vi "niFpga Discrete Transfer Function Direct.vi"(7 "reset":bool, 10 "FXP Transfer Function Model":T1={"Numerator"=[0.0, 0.0, 0.0, 0.0, 0.0, 0.0, 0.0, 0.0, 0.0], "Denominator"=[0.0, 0.0, 0.0, 0.0, 0.0, 0.0, 0.0, 0.0, 0.0], "Order"=0}, 11 "input u(k)":fxp<+/-,32,16>) -> (3 "output y(k)":fxp<+/-,32,16>)   [LabVIEW 2017]
doc: "Implements a fixed-point transfer function system model on an FPGA. Obtain this model by using the Discrete FP Transfer Function to FXP VI."
uses:
  <vilib>/rvi/Analysis/control/linear/templates/niFPGA FXP Transfer Function Model.ctl
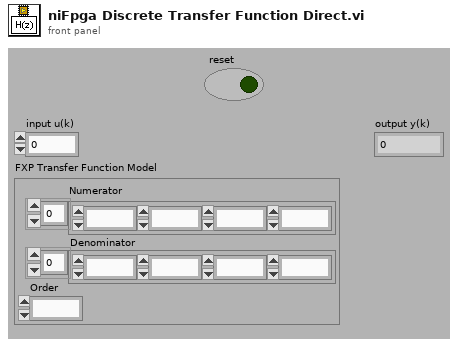
[diagram p1: front panel]
types:
  T1 = typedef "niFPGA FXP Transfer Function Model.ctl" = cluster{"Numerator":fxp<+/-,32,12>[], "Denominator":fxp<+/-,32,12>[], "Order":u8}
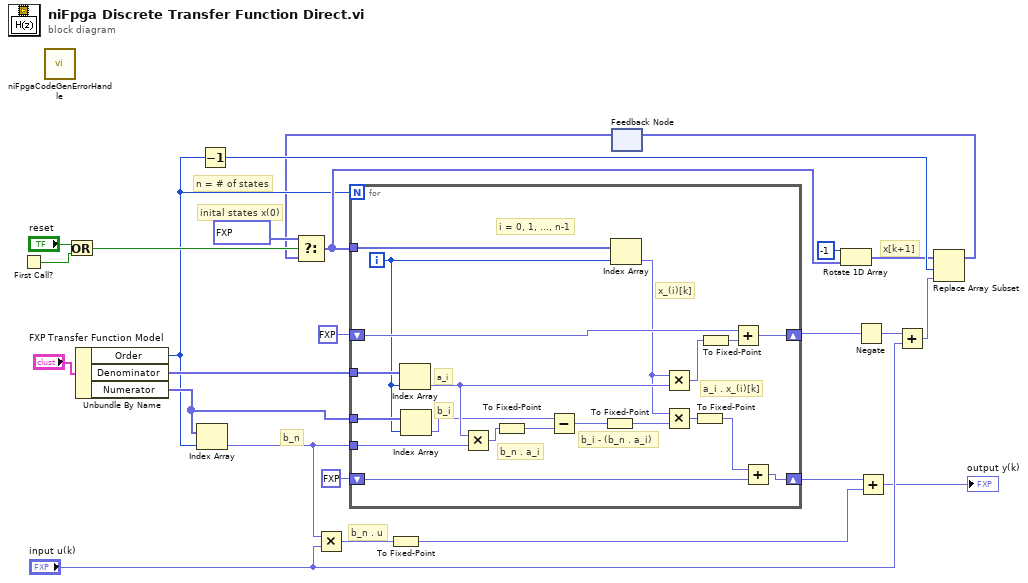
[diagram p0: block diagram]
diagram:
  # "b_n . u"
  # "b_n"
  # "x[k+1]"
  # "n = # of states"
  # "inital states x(0)"
  n1 = First Call?() -> (First Call?: T/F=w24:bool)
  n2 = call <vilib>:"niFpgaCodeGenErrorHandle.vi"() -> ()  [unwired: 1 in]
  n3 = Or(x="reset", y=w24) -> (x .or. y?=w23:bool)
  n4 = Unbundle By Name("FXP Transfer Function Model") -> ("Order"=w13:u8, "Denominator"=w14:fxp<+/-,32,12>[], "Numerator"=w19:fxp<+/-,32,12>[])
  n5 = Index Array(array=w19, index=w13) -> (element=w20:fxp<+/-,32,12>)
  n6 = Decrement(x=w13) -> (x-1=w17:u8)
  n7 = Multiply(x=w20, y="input u(k)") -> (x*y=w4:fxp<+/-,64,28>)
  n8 = To Fixed-Point(number=w4) -> (fixed-point=w3:fxp<+/-,32,16>)  [unwired: 1 in]
  n9 = feedback #1() -> (w12:fxp<+/-,32,16>[])  [unwired: 1 in]
  n10 = Select(t=fxp<+/-,32,16>[] [0.0, 0.0, 0.0, 0.0, 0.0, 0.0, 0.0, 0.0, 0.0] ("initialized array"), s=w23, f=w12) -> (s? t:f=w16:fxp<+/-,32,16>[])
  n11 = for {
    N: w13 -> [_]
    tunnel: w14 -> [w39]
    shift-right: [w44] -> w10
    shift-left: fxp<+/-,32,16> 0.0 ("element") -> [w45]
    tunnel: w19 -> [w38]
    tunnel: w20 -> [w43]
    shift-right: [w42] -> w7
    shift-left: fxp<+/-,32,16> 0.0 ("element") -> [w41]
    tunnel: w16 -> [w34]
    i -> [w36]
    # "i = 0, 1, ..., n-1"
    # "x_(i)[k]"
    # "b_i - (b_n . a_i)"
    # "b_n . a_i"
    # "b_i"
    # "a_i . x_(i)[k]"
    # "a_i"
    n12 = Index Array(array=w39, index=w36) -> (element=w40:fxp<+/-,32,12>)
    n13 = Index Array(array=w38, index=w36) -> (element=w37:fxp<+/-,32,12>)
    n14 = Multiply(x=w40, y=w43) -> (x*y=w33:fxp<+/-,64,24>)
    n15 = To Fixed-Point(number=w33) -> (fixed-point=w32:fxp<+/-,32,12>)  [unwired: 1 in]
    n16 = Subtract(x=w37, y=w32) -> (x-y=w31:fxp<+/-,33,13>)
    n17 = To Fixed-Point(number=w31) -> (fixed-point=w30:fxp<+/-,32,12>)  [unwired: 1 in]
    n18 = Index Array(array=w34, index=w36) -> (element=w35:fxp<+/-,32,16>)
    n19 = Multiply(x=w35, y=w40) -> (x*y=w27:fxp<+/-,64,28>)
    n20 = Multiply(x=w35, y=w30) -> (x*y=w29:fxp<+/-,64,28>)
    n21 = To Fixed-Point(number=w29) -> (fixed-point=w28:fxp<+/-,32,16>)  [unwired: 1 in]
    n22 = To Fixed-Point(number=w27) -> (fixed-point=w26:fxp<+/-,32,16>)  [unwired: 1 in]
    n23 = Add(x=w45, y=w26) -> (x+y=w44:fxp<+/-,32,16>)
    n24 = Add(x=w28, y=w41) -> (x+y=w42:fxp<+/-,32,16>)
  }
  n25 = Rotate 1D Array(1:w16, 2:-1 ("n")) -> (0:w1:fxp<+/-,32,16>[])
  n26 = Negate(x=w10) -> (-x=w9:fxp<+/-,33,17>)
  n27 = Add(x=w7, y=w3) -> (x+y=→"output y(k)":fxp<+/-,32,16>)
  n28 = Add(x=w9, y="input u(k)") -> (x+y=w8:fxp<+/-,32,16>)
  n29 = Replace Array Subset(array=w1, new element=w8, index=w17) -> (w11:fxp<+/-,32,16>[])
  n30 = feedback-in #1(w11) -> ()
